vi "Voltages_2_U16.vi"(0 "Voltages":dbl[][](array[numeric])) -> (1 "Scale and Offset":T1(array[cluster]), 2 "U16 data":u16[][](array[numeric]))   [LabVIEW 2010]
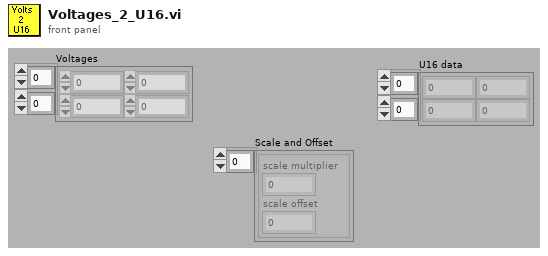
[diagram p1: front panel]
types:
  T1 = cluster{"scale multiplier":dbl, "scale offset":dbl}[]
  T2 = cluster{"scale multiplier":dbl, "scale offset":dbl}
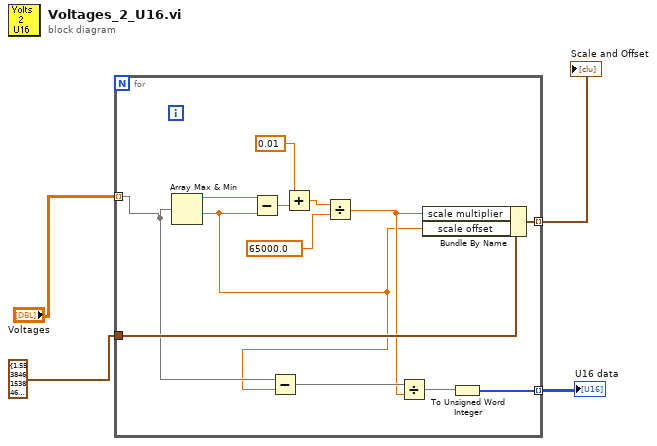
[diagram p0: block diagram]
diagram:
  n1 = for {
    tunnel: T2 {"scale multiplier"=1.553846153846154e-05, "scale offset"=1.0} -> [w17]
    tunnel: [w16] -> w3 mode=indexing
    tunnel: [w13] -> w2 mode=indexing
    tunnel: "Voltages" -> [w9] mode=indexing
    n2 = Array Max & Min(array=w9) -> (max value=w15:dbl, min value=w5:dbl)  [unwired: 2 out]
    n3 = Subtract(x=w15, y=w5) -> (x-y=w8:dbl)
    n4 = Subtract(x=w9, y=w5) -> (x-y=w11:dbl[])
    n5 = Add(x=0.01, y=w8) -> (x+y=w7:dbl)
    n6 = Divide(x=w7, y=65000.0) -> (x/y=w10:dbl)
    n7 = Divide(x=w11, y=w10) -> (x/y=w14:dbl[])
    n8 = Bundle By Name(cluster=w17, "scale multiplier"=w10, "scale offset"=w5) -> (w16:T2)
    n9 = To Unsigned Word Integer(number=w14) -> (unsigned 16bit integer=w13:u16[])
  }
  "Scale and Offset" <- w3
  "U16 data" <- w2
